vi "Write Y Scale.vi"(5 "Y scale":refnum<class "GraphScale.lvclass">, 9 "GraphChart in":refnum<class "GraphChart.lvclass">) -> (3 "GraphChart out":refnum<class "GraphChart.lvclass">)   [LabVIEW 2014, in "GraphChart.lvclass"]
uses:
  GraphChart.lvclass
  GraphScale/GraphScale.lvclass
  GraphChart.lvclass/GraphChart.ctl
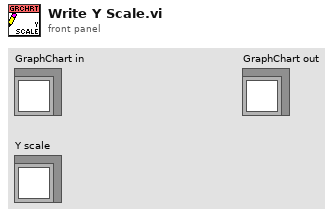
[diagram p1: front panel]
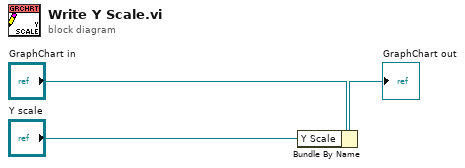
[diagram p0: block diagram]
diagram:
  n1 = Bundle By Name(cluster="GraphChart in", "Y Scale"="Y scale") -> (→"GraphChart out":refnum<class "GraphChart.lvclass">)
